vi "Create.vi"(8 "error in (no error)":errorcluster, 10 "GPIO":T1=-1) -> (0 "error out":errorcluster, 3 "PWM out":refnum<class "PWM.lvclass">)   [LabVIEW 2020, in "CTI.lvlib" / "PWM.lvclass"]
uses:
  PWM.lvclass
  GPIO Number.ctl
  PWM.lvclass/PWM.ctl
  CTI.lvlib
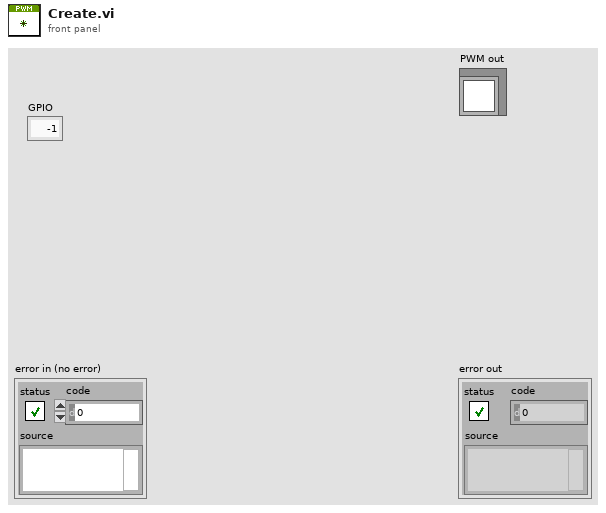
[diagram p1: front panel]
types:
  T1 = typedef "CTI.lvlib/GPIO Number.ctl" = i8
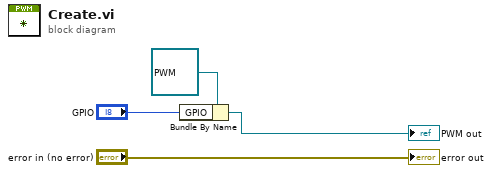
[diagram p0: block diagram]
diagram:
  n1 = Bundle By Name(cluster=refnum<class "PWM.lvclass"> refnum ("PWM in"), "GPIO"="GPIO") -> (→"PWM out":refnum<class "PWM.lvclass">)
  "error out" <- "error in (no error)"
